vi "New cRIO Health Alert.vi"(8 "error in (no error)":errorcluster, 11 "Alert (Last index value)":bool[](array[boolean])) -> (0 "error out":errorcluster)   [LabVIEW 2018]
doc: "This subVI enqueues the named action in to the communications queue along with the input data."
uses:
  Private Controls/Module Action.ctl
  RT - Instrument IO.lvlib
  Private Controls/Module Data.ctl
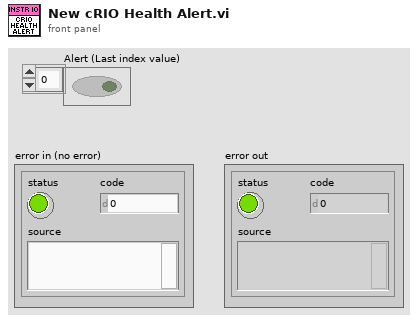
[diagram p1: front panel]
types:
  T1 = typedef "RT - Instrument IO.lvlib/Module Data.ctl" = cluster{"Data":variant, "Action":T2}
  T2 = typedef "RT - Instrument IO.lvlib/Module Action.ctl" = enum16{"Init", "Error", "Exit", "Timeout", "StartStop Acquisition", "Write 02-06-9265 Vals (AO)", "Write 00-04-9265 Vals (AO)", "Write 02-00-9485 Vals (DO)", "Write 02-01-9485 Vals (DO)", "Set APU&ECU Cntrls", "Set Bleed-Fuel-ECS Cntrls", "Loop Set Bleed-Fuel-ECS Cntrls", "Set ECS Demnd Cluster", "Set Fuel Pres Regltr", "Set Overspeed Thresholds", "Write Single 02-00-9485 Chann", "Write Single 02-01-9485 Chann", "Write Single 00-04-9265 Chann", "Set Sample Rate", "ESTOP", "New cRIO Health Alert"}
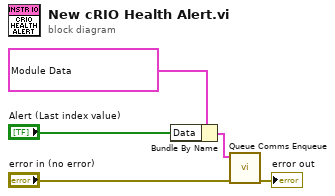
[diagram p0: block diagram]
diagram:
  n1 = Bundle By Name(cluster=T1 {"Data"=variant, "Action"=enum."New cRIO Health Alert"} ("element"), "Data"="Alert (Last index value)") -> (w5:T1)
  n2 = call "Queue Comms Enqueue.vi"("error in (no error)"="error in (no error)", "element"=w5) -> ("error out"=→"error out":errorcluster)  [unwired: 9 in]
